vi "IO.vi"() -> ()   [LabVIEW 2019]
uses:
  <vilib>/LabVIEW Targets/FPGA/RIO/BlueMoonOnboardIO/nicrio_cRIO-BlueMoonOnboardAi_TerminalMod.ctl
  <vilib>/LabVIEW Targets/FPGA/RIO/BlueMoonOnboardIO/nicrio_cRIO-BlueMoonOnboardAi_VoltageRange.ctl
  <vilib>/rvi/Emulation/niFpgaGetClockAttributes.vi
  <vilib>/rvi/Emulation/niFpgaSctlEmulationGetInTimedLoop.vi
  <vilib>/rvi/Emulation/niFpgaEmulationReportErrorSimple.vi
  <vilib>/rvi/eio/common/nirviEmuTemplateMethod_errors.vi
  <vilib>/rvi/eio/common/nirviEmuTemplatePropertySet_noerrors.vi
  <vilib>/rvi/Emulation/niFpgaCriticalErrorInLSC.vi
  <vilib>/eio/EIONode/EIONode.xnode
  <vilib>/eio/EIOMethodNode/EIOMethodNode.xnode
  <vilib>/eio/EIOPropertyNode/EIOPropertyNode.xnode
  <vilib>/rvi/eio/common/nirviEmuTemplatePropertyGet_errors.vi
  <vilib>/rvi/eio/common/nirviEmuTemplatePropertyGet_noerrors.vi
  <vilib>/rvi/eio/common/nirviEmuTemplatePropertySet_errors.vi
panel:
  in  "outputAO3":fxp<+/-,20,5>
  in  "outputAO2":fxp<+/-,20,5>
  in  "outputAO1":fxp<+/-,20,5>
  in  "outputAO0":fxp<+/-,20,5>
  in  "rangeAI15":T1 items=["+/- 10V", "+/- 5V", "+/- 2V", "+/- 1V"]
  in  "modeAI15":T2=1 items=["DIFF", "RSE"]
  out "inputAI15":fxp<+/-,24,5>
  in  "rangeAI14":T1 items=["+/- 10V", "+/- 5V", "+/- 2V", "+/- 1V"]
  in  "modeAI14":T2=1 items=["DIFF", "RSE"]
  out "inputAI14":fxp<+/-,24,5>
  in  "rangeAI13":T1 items=["+/- 10V", "+/- 5V", "+/- 2V", "+/- 1V"]
  in  "modeAI13":T2=1 items=["DIFF", "RSE"]
  out "inputAI13":fxp<+/-,24,5>
  in  "rangeAI12":T1 items=["+/- 10V", "+/- 5V", "+/- 2V", "+/- 1V"]
  in  "modeAI12":T2=1 items=["DIFF", "RSE"]
  out "inputAI12":fxp<+/-,24,5>
  in  "rangeAI11":T1 items=["+/- 10V", "+/- 5V", "+/- 2V", "+/- 1V"]
  in  "modeAI11":T2=1 items=["DIFF", "RSE"]
  out "inputAI11":fxp<+/-,24,5>
  in  "rangeAI10":T1 items=["+/- 10V", "+/- 5V", "+/- 2V", "+/- 1V"]
  in  "modeAI10":T2=1 items=["DIFF", "RSE"]
  out "inputAI10":fxp<+/-,24,5>
  in  "rangeAI9":T1 items=["+/- 10V", "+/- 5V", "+/- 2V", "+/- 1V"]
  in  "modeAI9":T2=1 items=["DIFF", "RSE"]
  out "inputAI9":fxp<+/-,24,5>
  in  "rangeAI8":T1 items=["+/- 10V", "+/- 5V", "+/- 2V", "+/- 1V"]
  in  "modeAI8":T2=1 items=["DIFF", "RSE"]
  out "inputAI8":fxp<+/-,24,5>
  in  "rangeAI7":T1 items=["+/- 10V", "+/- 5V", "+/- 2V", "+/- 1V"]
  in  "modeAI7":T2=1 items=["DIFF", "RSE"]
  out "inputAI7":fxp<+/-,24,5>
  in  "rangeAI6":T1 items=["+/- 10V", "+/- 5V", "+/- 2V", "+/- 1V"]
  in  "modeAI6":T2=1 items=["DIFF", "RSE"]
  out "inputAI6":fxp<+/-,24,5>
  in  "rangeAI5":T1 items=["+/- 10V", "+/- 5V", "+/- 2V", "+/- 1V"]
  in  "modeAI5":T2=1 items=["DIFF", "RSE"]
  out "inputAI5":fxp<+/-,24,5>
  in  "rangeAI4":T1 items=["+/- 10V", "+/- 5V", "+/- 2V", "+/- 1V"]
  in  "modeAI4":T2=1 items=["DIFF", "RSE"]
  out "inputAI4":fxp<+/-,24,5>
  in  "rangeAI3":T1 items=["+/- 10V", "+/- 5V", "+/- 2V", "+/- 1V"]
  in  "modeAI3":T2=1 items=["DIFF", "RSE"]
  out "inputAI3":fxp<+/-,24,5>
  in  "rangeAI2":T1 items=["+/- 10V", "+/- 5V", "+/- 2V", "+/- 1V"]
  in  "modeAI2":T2=1 items=["DIFF", "RSE"]
  out "inputAI2":fxp<+/-,24,5>
  in  "rangeAI1":T1 items=["+/- 10V", "+/- 5V", "+/- 2V", "+/- 1V"]
  in  "modeAI1":T2=1 items=["DIFF", "RSE"]
  out "inputAI1":fxp<+/-,24,5>
  in  "rangeAI0":T1 items=["+/- 10V", "+/- 5V", "+/- 2V", "+/- 1V"]
  in  "modeAI0":T2=1 items=["DIFF", "RSE"]
  out "inputAI0":fxp<+/-,24,5>
  in  "outDIO27":bool
  in  "outputEnableDIO27":bool
  out "inDIO27":bool
  in  "outDIO26":bool
  in  "outputEnableDIO26":bool
  out "inDIO26":bool
  in  "outDIO25":bool
  in  "outputEnableDIO25":bool
  out "inDIO25":bool
  in  "outDIO24":bool
  in  "outputEnableDIO24":bool
  out "inDIO24":bool
  in  "outDIO23":bool
  in  "outputEnableDIO23":bool
  out "inDIO23":bool
  in  "outDIO22":bool
  in  "outputEnableDIO22":bool
  out "inDIO22":bool
  in  "outDIO21":bool
  in  "outputEnableDIO21":bool
  out "inDIO21":bool
  in  "outDIO20":bool
  in  "outputEnableDIO20":bool
  out "inDIO20":bool
  in  "outDIO19":bool
  in  "outputEnableDIO19":bool
  out "inDIO19":bool
  in  "outDIO18":bool
  in  "outputEnableDIO18":bool
  out "inDIO18":bool
  in  "outDIO17":bool
  in  "outputEnableDIO17":bool
  out "inDIO17":bool
  in  "outDIO16":bool
  in  "outputEnableDIO16":bool
  out "inDIO16":bool
  in  "outDIO15":bool
  in  "outputEnableDIO15":bool
  out "inDIO15":bool
  in  "outDIO14":bool
  in  "outputEnableDIO14":bool
  out "inDIO14":bool
  in  "outDIO13":bool
  in  "outputEnableDIO13":bool
  out "inDIO13":bool
  in  "outDIO12":bool
  in  "outputEnableDIO12":bool
  out "inDIO12":bool
  in  "outDIO11":bool
  in  "outputEnableDIO11":bool
  out "inDIO11":bool
  in  "outDIO10":bool
  in  "outputEnableDIO10":bool
  out "inDIO10":bool
  in  "outDIO9":bool
  in  "outputEnableDIO9":bool
  out "inDIO9":bool
  in  "outDIO8":bool
  in  "outputEnableDIO8":bool
  out "inDIO8":bool
  in  "outDIO7":bool
  in  "outputEnableDIO7":bool
  out "inDIO7":bool
  in  "outDIO6":bool
  in  "outputEnableDIO6":bool
  out "inDIO6":bool
  in  "outDIO5":bool
  in  "outputEnableDIO5":bool
  out "inDIO5":bool
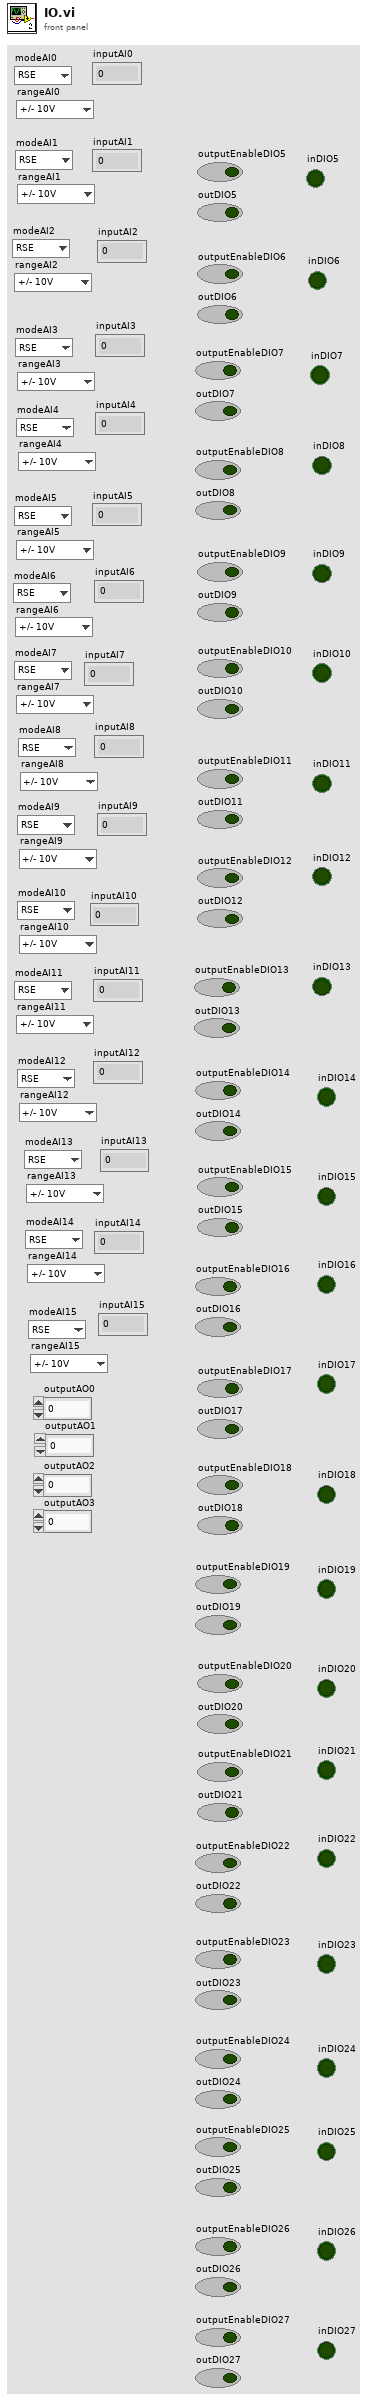
[diagram p1: front panel]
types:
  T1 = typedef "nicrio_cRIO-BlueMoonOnboardAi_VoltageRange.ctl" = u8
  T2 = typedef "nicrio_cRIO-BlueMoonOnboardAi_TerminalMod.ctl" = u8
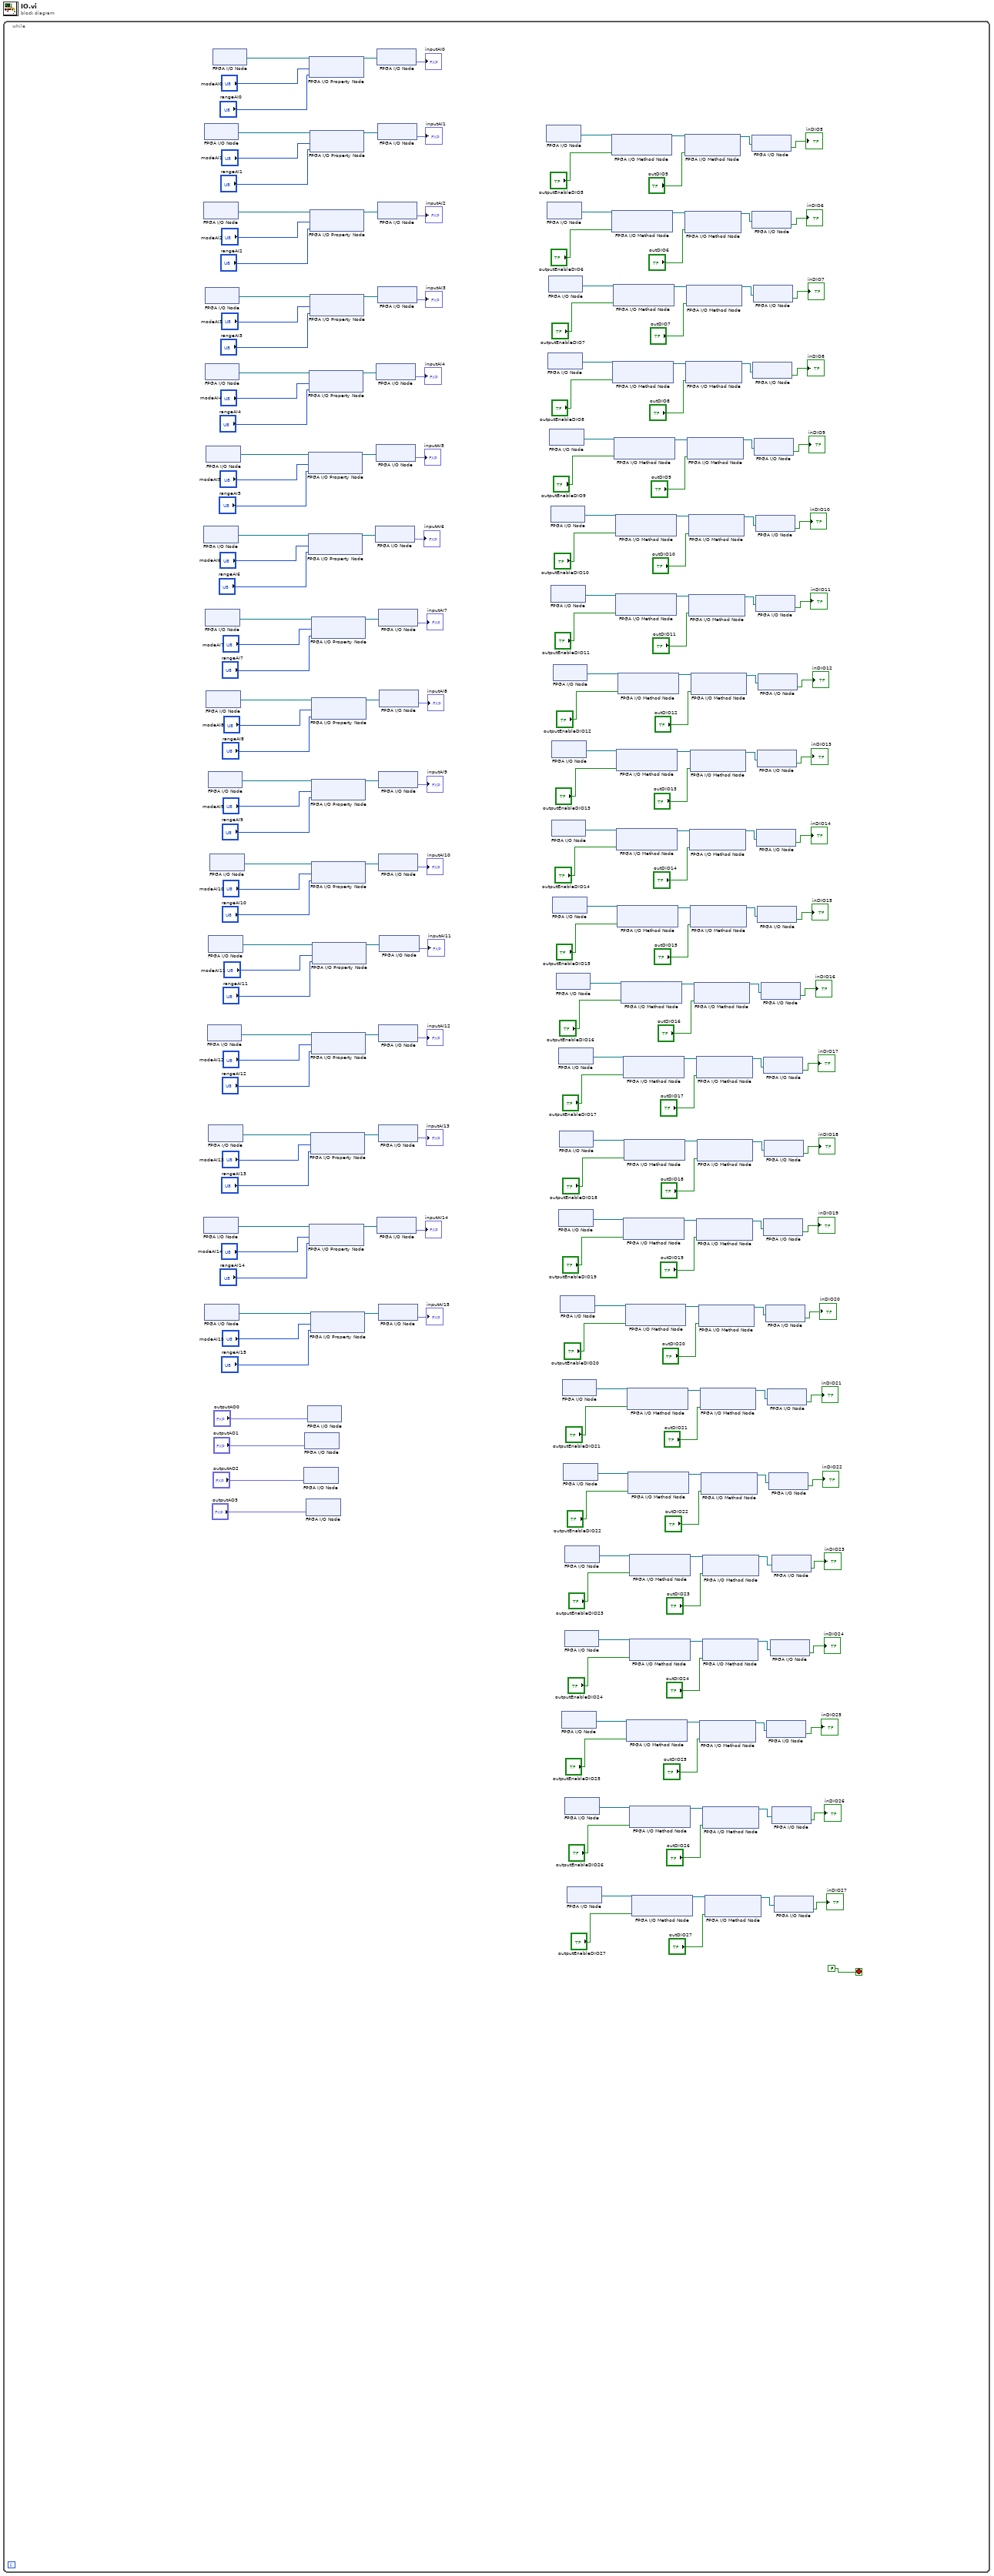
[diagram p0: block diagram]
diagram:
  n1 = while {
    stop <- FALSE stop-if-true
    n2 = xnode "FPGA I/O Node"() -> ("FPGA I/O Out"=w71:refnum<k21>)  [unwired: 1 in, 1 out]
    n3 = xnode "FPGA I/O Node"() -> ("FPGA I/O Out"=w51:refnum<k21>)  [unwired: 1 in, 1 out]
    n4 = xnode "FPGA I/O Node"() -> ("FPGA I/O Out"=w11:refnum<k21>)  [unwired: 1 in, 1 out]
    n5 = xnode "FPGA I/O Node"() -> ("FPGA I/O Out"=w76:refnum<k21>)  [unwired: 1 in, 1 out]
    n6 = xnode "FPGA I/O Node"() -> ("FPGA I/O Out"=w6:refnum<k21>)  [unwired: 1 in, 1 out]
    n7 = xnode "FPGA I/O Node"() -> ("FPGA I/O Out"=w66:refnum<k21>)  [unwired: 1 in, 1 out]
    n8 = xnode "FPGA I/O Node"() -> ("FPGA I/O Out"=w61:refnum<k21>)  [unwired: 1 in, 1 out]
    n9 = xnode "FPGA I/O Node"() -> ("FPGA I/O Out"=w46:refnum<k21>)  [unwired: 1 in, 1 out]
    n10 = xnode "FPGA I/O Node"() -> ("FPGA I/O Out"=w41:refnum<k21>)  [unwired: 1 in, 1 out]
    n11 = xnode "FPGA I/O Node"() -> ("FPGA I/O Out"=w56:refnum<k21>)  [unwired: 1 in, 1 out]
    n12 = xnode "FPGA I/O Node"() -> ("FPGA I/O Out"=w21:refnum<k21>)  [unwired: 1 in, 1 out]
    n13 = xnode "FPGA I/O Node"() -> ("FPGA I/O Out"=w36:refnum<k21>)  [unwired: 1 in, 1 out]
    n14 = xnode "FPGA I/O Node"() -> ("FPGA I/O Out"=w26:refnum<k21>)  [unwired: 1 in, 1 out]
    n15 = xnode "FPGA I/O Node"() -> ("FPGA I/O Out"=w16:refnum<k21>)  [unwired: 1 in, 1 out]
    n16 = xnode "FPGA I/O Node"() -> ("FPGA I/O Out"=w31:refnum<k21>)  [unwired: 1 in, 1 out]
    n17 = xnode "FPGA I/O Node"() -> ("FPGA I/O Out"=w85:refnum<k21>)  [unwired: 1 in, 1 out]
    n18 = xnode "FPGA I/O Node"("AO2"="outputAO2") -> ()  [unwired: 1 in, 1 out]
    n19 = xnode "FPGA I/O Node"("AO1"="outputAO1") -> ()  [unwired: 1 in, 1 out]
    n20 = xnode "FPGA I/O Node"("AO3"="outputAO3") -> ()  [unwired: 1 in, 1 out]
    n21 = xnode "FPGA I/O Node"("AO0"="outputAO0") -> ()  [unwired: 1 in, 1 out]
    n22 = xnode "FPGA I/O Property Node"("FPGA I/O In"=w51, "Terminal Mode"="modeAI6", "Voltage Range"="rangeAI6") -> ("FPGA I/O Out"=w55:refnum<k21>)
    n23 = xnode "FPGA I/O Property Node"("FPGA I/O In"=w56, "Terminal Mode"="modeAI5", "Voltage Range"="rangeAI5") -> ("FPGA I/O Out"=w60:refnum<k21>)
    n24 = xnode "FPGA I/O Property Node"("FPGA I/O In"=w61, "Terminal Mode"="modeAI4", "Voltage Range"="rangeAI4") -> ("FPGA I/O Out"=w65:refnum<k21>)
    n25 = xnode "FPGA I/O Property Node"("FPGA I/O In"=w85, "Terminal Mode"="modeAI0", "Voltage Range"="rangeAI0") -> ("FPGA I/O Out"=w84:refnum<k21>)
    n26 = xnode "FPGA I/O Property Node"("FPGA I/O In"=w11, "Terminal Mode"="modeAI14", "Voltage Range"="rangeAI14") -> ("FPGA I/O Out"=w15:refnum<k21>)
    n27 = xnode "FPGA I/O Property Node"("FPGA I/O In"=w76, "Terminal Mode"="modeAI1", "Voltage Range"="rangeAI1") -> ("FPGA I/O Out"=w80:refnum<k21>)
    n28 = xnode "FPGA I/O Property Node"("FPGA I/O In"=w71, "Terminal Mode"="modeAI2", "Voltage Range"="rangeAI2") -> ("FPGA I/O Out"=w72:refnum<k21>)
    n29 = xnode "FPGA I/O Property Node"("FPGA I/O In"=w66, "Terminal Mode"="modeAI3", "Voltage Range"="rangeAI3") -> ("FPGA I/O Out"=w70:refnum<k21>)
    n30 = xnode "FPGA I/O Property Node"("FPGA I/O In"=w16, "Terminal Mode"="modeAI13", "Voltage Range"="rangeAI13") -> ("FPGA I/O Out"=w20:refnum<k21>)
    n31 = xnode "FPGA I/O Property Node"("FPGA I/O In"=w6, "Terminal Mode"="modeAI15", "Voltage Range"="rangeAI15") -> ("FPGA I/O Out"=w10:refnum<k21>)
    n32 = xnode "FPGA I/O Property Node"("FPGA I/O In"=w46, "Terminal Mode"="modeAI7", "Voltage Range"="rangeAI7") -> ("FPGA I/O Out"=w50:refnum<k21>)
    n33 = xnode "FPGA I/O Property Node"("FPGA I/O In"=w36, "Terminal Mode"="modeAI9", "Voltage Range"="rangeAI9") -> ("FPGA I/O Out"=w40:refnum<k21>)
    n34 = xnode "FPGA I/O Property Node"("FPGA I/O In"=w31, "Terminal Mode"="modeAI10", "Voltage Range"="rangeAI10") -> ("FPGA I/O Out"=w35:refnum<k21>)
    n35 = xnode "FPGA I/O Property Node"("FPGA I/O In"=w21, "Terminal Mode"="modeAI12", "Voltage Range"="rangeAI12") -> ("FPGA I/O Out"=w25:refnum<k21>)
    n36 = xnode "FPGA I/O Property Node"("FPGA I/O In"=w41, "Terminal Mode"="modeAI8", "Voltage Range"="rangeAI8") -> ("FPGA I/O Out"=w45:refnum<k21>)
    n37 = xnode "FPGA I/O Property Node"("FPGA I/O In"=w26, "Terminal Mode"="modeAI11", "Voltage Range"="rangeAI11") -> ("FPGA I/O Out"=w30:refnum<k21>)
    n38 = xnode "FPGA I/O Node"("FPGA I/O In"=w55) -> ("I/O Item"=→"inputAI6":fxp<+/-,24,5>)  [unwired: 1 out]
    n39 = xnode "FPGA I/O Node"("FPGA I/O In"=w60) -> ("I/O Item"=→"inputAI5":fxp<+/-,24,5>)  [unwired: 1 out]
    n40 = xnode "FPGA I/O Node"("FPGA I/O In"=w65) -> ("I/O Item"=→"inputAI4":fxp<+/-,24,5>)  [unwired: 1 out]
    n41 = xnode "FPGA I/O Node"("FPGA I/O In"=w84) -> ("I/O Item"=→"inputAI0":fxp<+/-,24,5>)  [unwired: 1 out]
    n42 = xnode "FPGA I/O Node"("FPGA I/O In"=w15) -> ("I/O Item"=→"inputAI14":fxp<+/-,24,5>)  [unwired: 1 out]
    n43 = xnode "FPGA I/O Node"("FPGA I/O In"=w80) -> ("I/O Item"=→"inputAI1":fxp<+/-,24,5>)  [unwired: 1 out]
    n44 = xnode "FPGA I/O Node"("FPGA I/O In"=w72) -> ("I/O Item"=→"inputAI2":fxp<+/-,24,5>)  [unwired: 1 out]
    n45 = xnode "FPGA I/O Node"("FPGA I/O In"=w70) -> ("I/O Item"=→"inputAI3":fxp<+/-,24,5>)  [unwired: 1 out]
    n46 = xnode "FPGA I/O Node"("FPGA I/O In"=w20) -> ("I/O Item"=→"inputAI13":fxp<+/-,24,5>)  [unwired: 1 out]
    n47 = xnode "FPGA I/O Node"("FPGA I/O In"=w10) -> ("I/O Item"=→"inputAI15":fxp<+/-,24,5>)  [unwired: 1 out]
    n48 = xnode "FPGA I/O Node"("FPGA I/O In"=w50) -> ("I/O Item"=→"inputAI7":fxp<+/-,24,5>)  [unwired: 1 out]
    n49 = xnode "FPGA I/O Node"("FPGA I/O In"=w40) -> ("I/O Item"=→"inputAI9":fxp<+/-,24,5>)  [unwired: 1 out]
    n50 = xnode "FPGA I/O Node"("FPGA I/O In"=w35) -> ("I/O Item"=→"inputAI10":fxp<+/-,24,5>)  [unwired: 1 out]
    n51 = xnode "FPGA I/O Node"("FPGA I/O In"=w25) -> ("I/O Item"=→"inputAI12":fxp<+/-,24,5>)  [unwired: 1 out]
    n52 = xnode "FPGA I/O Node"("FPGA I/O In"=w45) -> ("I/O Item"=→"inputAI8":fxp<+/-,24,5>)  [unwired: 1 out]
    n53 = xnode "FPGA I/O Node"("FPGA I/O In"=w30) -> ("I/O Item"=→"inputAI11":fxp<+/-,24,5>)  [unwired: 1 out]
    n54 = xnode "FPGA I/O Node"() -> ("FPGA I/O Out"=w223:refnum<k21>)  [unwired: 1 in, 1 out]
    n55 = xnode "FPGA I/O Node"() -> ("FPGA I/O Out"=w212:refnum<k21>)  [unwired: 1 in, 1 out]
    n56 = xnode "FPGA I/O Node"() -> ("FPGA I/O Out"=w205:refnum<k21>)  [unwired: 1 in, 1 out]
    n57 = xnode "FPGA I/O Node"() -> ("FPGA I/O Out"=w211:refnum<k21>)  [unwired: 1 in, 1 out]
    n58 = xnode "FPGA I/O Node"() -> ("FPGA I/O Out"=w199:refnum<k21>)  [unwired: 1 in, 1 out]
    n59 = xnode "FPGA I/O Node"() -> ("FPGA I/O Out"=w193:refnum<k21>)  [unwired: 1 in, 1 out]
    n60 = xnode "FPGA I/O Node"() -> ("FPGA I/O Out"=w187:refnum<k21>)  [unwired: 1 in, 1 out]
    n61 = xnode "FPGA I/O Node"() -> ("FPGA I/O Out"=w164:refnum<k21>)  [unwired: 1 in, 1 out]
    n62 = xnode "FPGA I/O Node"() -> ("FPGA I/O Out"=w175:refnum<k21>)  [unwired: 1 in, 1 out]
    n63 = xnode "FPGA I/O Node"() -> ("FPGA I/O Out"=w158:refnum<k21>)  [unwired: 1 in, 1 out]
    n64 = xnode "FPGA I/O Node"() -> ("FPGA I/O Out"=w176:refnum<k21>)  [unwired: 1 in, 1 out]
    n65 = xnode "FPGA I/O Node"() -> ("FPGA I/O Out"=w152:refnum<k21>)  [unwired: 1 in, 1 out]
    n66 = xnode "FPGA I/O Node"() -> ("FPGA I/O Out"=w146:refnum<k21>)  [unwired: 1 in, 1 out]
    n67 = xnode "FPGA I/O Node"() -> ("FPGA I/O Out"=w134:refnum<k21>)  [unwired: 1 in, 1 out]
    n68 = xnode "FPGA I/O Node"() -> ("FPGA I/O Out"=w140:refnum<k21>)  [unwired: 1 in, 1 out]
    n69 = xnode "FPGA I/O Node"() -> ("FPGA I/O Out"=w128:refnum<k21>)  [unwired: 1 in, 1 out]
    n70 = xnode "FPGA I/O Node"() -> ("FPGA I/O Out"=w98:refnum<k21>)  [unwired: 1 in, 1 out]
    n71 = xnode "FPGA I/O Node"() -> ("FPGA I/O Out"=w122:refnum<k21>)  [unwired: 1 in, 1 out]
    n72 = xnode "FPGA I/O Node"() -> ("FPGA I/O Out"=w116:refnum<k21>)  [unwired: 1 in, 1 out]
    n73 = xnode "FPGA I/O Node"() -> ("FPGA I/O Out"=w104:refnum<k21>)  [unwired: 1 in, 1 out]
    n74 = xnode "FPGA I/O Node"() -> ("FPGA I/O Out"=w110:refnum<k21>)  [unwired: 1 in, 1 out]
    n75 = xnode "FPGA I/O Node"() -> ("FPGA I/O Out"=w92:refnum<k21>)  [unwired: 1 in, 1 out]
    n76 = xnode "FPGA I/O Node"() -> ("FPGA I/O Out"=w86:refnum<k21>)  [unwired: 1 in, 1 out]
    n77 = xnode "FPGA I/O Method Node"("FPGA I/O In"=w223, "Enable"="outputEnableDIO5") -> ("FPGA I/O Out"=w222:refnum<k21>)
    n78 = xnode "FPGA I/O Method Node"("FPGA I/O In"=w212, "Enable"="outputEnableDIO6") -> ("FPGA I/O Out"=w213:refnum<k21>)
    n79 = xnode "FPGA I/O Method Node"("FPGA I/O In"=w205, "Enable"="outputEnableDIO8") -> ("FPGA I/O Out"=w204:refnum<k21>)
    n80 = xnode "FPGA I/O Method Node"("FPGA I/O In"=w211, "Enable"="outputEnableDIO7") -> ("FPGA I/O Out"=w210:refnum<k21>)
    n81 = xnode "FPGA I/O Method Node"("FPGA I/O In"=w199, "Enable"="outputEnableDIO9") -> ("FPGA I/O Out"=w198:refnum<k21>)
    n82 = xnode "FPGA I/O Method Node"("FPGA I/O In"=w193, "Enable"="outputEnableDIO10") -> ("FPGA I/O Out"=w192:refnum<k21>)
    n83 = xnode "FPGA I/O Method Node"("FPGA I/O In"=w187, "Enable"="outputEnableDIO11") -> ("FPGA I/O Out"=w186:refnum<k21>)
    n84 = xnode "FPGA I/O Method Node"("FPGA I/O In"=w164, "Enable"="outputEnableDIO14") -> ("FPGA I/O Out"=w165:refnum<k21>)
    n85 = xnode "FPGA I/O Method Node"("FPGA I/O In"=w175, "Enable"="outputEnableDIO13") -> ("FPGA I/O Out"=w174:refnum<k21>)
    n86 = xnode "FPGA I/O Method Node"("FPGA I/O In"=w158, "Enable"="outputEnableDIO15") -> ("FPGA I/O Out"=w159:refnum<k21>)
    n87 = xnode "FPGA I/O Method Node"("FPGA I/O In"=w176, "Enable"="outputEnableDIO12") -> ("FPGA I/O Out"=w177:refnum<k21>)
    n88 = xnode "FPGA I/O Method Node"("FPGA I/O In"=w152, "Enable"="outputEnableDIO16") -> ("FPGA I/O Out"=w153:refnum<k21>)
    n89 = xnode "FPGA I/O Method Node"("FPGA I/O In"=w146, "Enable"="outputEnableDIO17") -> ("FPGA I/O Out"=w147:refnum<k21>)
    n90 = xnode "FPGA I/O Method Node"("FPGA I/O In"=w134, "Enable"="outputEnableDIO19") -> ("FPGA I/O Out"=w135:refnum<k21>)
    n91 = xnode "FPGA I/O Method Node"("FPGA I/O In"=w140, "Enable"="outputEnableDIO18") -> ("FPGA I/O Out"=w141:refnum<k21>)
    n92 = xnode "FPGA I/O Method Node"("FPGA I/O In"=w128, "Enable"="outputEnableDIO20") -> ("FPGA I/O Out"=w129:refnum<k21>)
    n93 = xnode "FPGA I/O Method Node"("FPGA I/O In"=w98, "Enable"="outputEnableDIO25") -> ("FPGA I/O Out"=w99:refnum<k21>)
    n94 = xnode "FPGA I/O Method Node"("FPGA I/O In"=w122, "Enable"="outputEnableDIO21") -> ("FPGA I/O Out"=w123:refnum<k21>)
    n95 = xnode "FPGA I/O Method Node"("FPGA I/O In"=w116, "Enable"="outputEnableDIO22") -> ("FPGA I/O Out"=w117:refnum<k21>)
    n96 = xnode "FPGA I/O Method Node"("FPGA I/O In"=w104, "Enable"="outputEnableDIO24") -> ("FPGA I/O Out"=w105:refnum<k21>)
    n97 = xnode "FPGA I/O Method Node"("FPGA I/O In"=w110, "Enable"="outputEnableDIO23") -> ("FPGA I/O Out"=w111:refnum<k21>)
    n98 = xnode "FPGA I/O Method Node"("FPGA I/O In"=w92, "Enable"="outputEnableDIO26") -> ("FPGA I/O Out"=w93:refnum<k21>)
    n99 = xnode "FPGA I/O Method Node"("FPGA I/O In"=w86, "Enable"="outputEnableDIO27") -> ("FPGA I/O Out"=w87:refnum<k21>)
    n100 = xnode "FPGA I/O Method Node"("FPGA I/O In"=w222, "Data"="outDIO5") -> ("FPGA I/O Out"=w221:refnum<k21>)
    n101 = xnode "FPGA I/O Method Node"("FPGA I/O In"=w213, "Data"="outDIO6") -> ("FPGA I/O Out"=w214:refnum<k21>)
    n102 = xnode "FPGA I/O Method Node"("FPGA I/O In"=w204, "Data"="outDIO8") -> ("FPGA I/O Out"=w203:refnum<k21>)
    n103 = xnode "FPGA I/O Method Node"("FPGA I/O In"=w210, "Data"="outDIO7") -> ("FPGA I/O Out"=w209:refnum<k21>)
    n104 = xnode "FPGA I/O Method Node"("FPGA I/O In"=w198, "Data"="outDIO9") -> ("FPGA I/O Out"=w197:refnum<k21>)
    n105 = xnode "FPGA I/O Method Node"("FPGA I/O In"=w192, "Data"="outDIO10") -> ("FPGA I/O Out"=w191:refnum<k21>)
    n106 = xnode "FPGA I/O Method Node"("FPGA I/O In"=w186, "Data"="outDIO11") -> ("FPGA I/O Out"=w185:refnum<k21>)
    n107 = xnode "FPGA I/O Method Node"("FPGA I/O In"=w165, "Data"="outDIO14") -> ("FPGA I/O Out"=w166:refnum<k21>)
    n108 = xnode "FPGA I/O Method Node"("FPGA I/O In"=w174, "Data"="outDIO13") -> ("FPGA I/O Out"=w173:refnum<k21>)
    n109 = xnode "FPGA I/O Method Node"("FPGA I/O In"=w159, "Data"="outDIO15") -> ("FPGA I/O Out"=w160:refnum<k21>)
    n110 = xnode "FPGA I/O Method Node"("FPGA I/O In"=w177, "Data"="outDIO12") -> ("FPGA I/O Out"=w178:refnum<k21>)
    n111 = xnode "FPGA I/O Method Node"("FPGA I/O In"=w153, "Data"="outDIO16") -> ("FPGA I/O Out"=w154:refnum<k21>)
    n112 = xnode "FPGA I/O Method Node"("FPGA I/O In"=w147, "Data"="outDIO17") -> ("FPGA I/O Out"=w148:refnum<k21>)
    n113 = xnode "FPGA I/O Method Node"("FPGA I/O In"=w135, "Data"="outDIO19") -> ("FPGA I/O Out"=w136:refnum<k21>)
    n114 = xnode "FPGA I/O Method Node"("FPGA I/O In"=w141, "Data"="outDIO18") -> ("FPGA I/O Out"=w142:refnum<k21>)
    n115 = xnode "FPGA I/O Method Node"("FPGA I/O In"=w129, "Data"="outDIO20") -> ("FPGA I/O Out"=w130:refnum<k21>)
    n116 = xnode "FPGA I/O Method Node"("FPGA I/O In"=w99, "Data"="outDIO25") -> ("FPGA I/O Out"=w100:refnum<k21>)
    n117 = xnode "FPGA I/O Method Node"("FPGA I/O In"=w123, "Data"="outDIO21") -> ("FPGA I/O Out"=w124:refnum<k21>)
    n118 = xnode "FPGA I/O Method Node"("FPGA I/O In"=w117, "Data"="outDIO22") -> ("FPGA I/O Out"=w118:refnum<k21>)
    n119 = xnode "FPGA I/O Method Node"("FPGA I/O In"=w105, "Data"="outDIO24") -> ("FPGA I/O Out"=w106:refnum<k21>)
    n120 = xnode "FPGA I/O Method Node"("FPGA I/O In"=w111, "Data"="outDIO23") -> ("FPGA I/O Out"=w112:refnum<k21>)
    n121 = xnode "FPGA I/O Method Node"("FPGA I/O In"=w93, "Data"="outDIO26") -> ("FPGA I/O Out"=w94:refnum<k21>)
    n122 = xnode "FPGA I/O Method Node"("FPGA I/O In"=w87, "Data"="outDIO27") -> ("FPGA I/O Out"=w88:refnum<k21>)
    n123 = xnode "FPGA I/O Node"("FPGA I/O In"=w221) -> ("I/O Item"=→"inDIO5":bool)  [unwired: 1 out]
    n124 = xnode "FPGA I/O Node"("FPGA I/O In"=w214) -> ("I/O Item"=→"inDIO6":bool)  [unwired: 1 out]
    n125 = xnode "FPGA I/O Node"("FPGA I/O In"=w203) -> ("I/O Item"=→"inDIO8":bool)  [unwired: 1 out]
    n126 = xnode "FPGA I/O Node"("FPGA I/O In"=w209) -> ("I/O Item"=→"inDIO7":bool)  [unwired: 1 out]
    n127 = xnode "FPGA I/O Node"("FPGA I/O In"=w197) -> ("I/O Item"=→"inDIO9":bool)  [unwired: 1 out]
    n128 = xnode "FPGA I/O Node"("FPGA I/O In"=w191) -> ("I/O Item"=→"inDIO10":bool)  [unwired: 1 out]
    n129 = xnode "FPGA I/O Node"("FPGA I/O In"=w185) -> ("I/O Item"=→"inDIO11":bool)  [unwired: 1 out]
    n130 = xnode "FPGA I/O Node"("FPGA I/O In"=w166) -> ("I/O Item"=→"inDIO14":bool)  [unwired: 1 out]
    n131 = xnode "FPGA I/O Node"("FPGA I/O In"=w173) -> ("I/O Item"=→"inDIO13":bool)  [unwired: 1 out]
    n132 = xnode "FPGA I/O Node"("FPGA I/O In"=w160) -> ("I/O Item"=→"inDIO15":bool)  [unwired: 1 out]
    n133 = xnode "FPGA I/O Node"("FPGA I/O In"=w178) -> ("I/O Item"=→"inDIO12":bool)  [unwired: 1 out]
    n134 = xnode "FPGA I/O Node"("FPGA I/O In"=w154) -> ("I/O Item"=→"inDIO16":bool)  [unwired: 1 out]
    n135 = xnode "FPGA I/O Node"("FPGA I/O In"=w148) -> ("I/O Item"=→"inDIO17":bool)  [unwired: 1 out]
    n136 = xnode "FPGA I/O Node"("FPGA I/O In"=w136) -> ("I/O Item"=→"inDIO19":bool)  [unwired: 1 out]
    n137 = xnode "FPGA I/O Node"("FPGA I/O In"=w142) -> ("I/O Item"=→"inDIO18":bool)  [unwired: 1 out]
    n138 = xnode "FPGA I/O Node"("FPGA I/O In"=w130) -> ("I/O Item"=→"inDIO20":bool)  [unwired: 1 out]
    n139 = xnode "FPGA I/O Node"("FPGA I/O In"=w100) -> ("I/O Item"=→"inDIO25":bool)  [unwired: 1 out]
    n140 = xnode "FPGA I/O Node"("FPGA I/O In"=w124) -> ("I/O Item"=→"inDIO21":bool)  [unwired: 1 out]
    n141 = xnode "FPGA I/O Node"("FPGA I/O In"=w118) -> ("I/O Item"=→"inDIO22":bool)  [unwired: 1 out]
    n142 = xnode "FPGA I/O Node"("FPGA I/O In"=w106) -> ("I/O Item"=→"inDIO24":bool)  [unwired: 1 out]
    n143 = xnode "FPGA I/O Node"("FPGA I/O In"=w112) -> ("I/O Item"=→"inDIO23":bool)  [unwired: 1 out]
    n144 = xnode "FPGA I/O Node"("FPGA I/O In"=w94) -> ("I/O Item"=→"inDIO26":bool)  [unwired: 1 out]
    n145 = xnode "FPGA I/O Node"("FPGA I/O In"=w88) -> ("I/O Item"=→"inDIO27":bool)  [unwired: 1 out]
  }
